vi "read creates channels.vi"(8 "error in":errorcluster, 11 "module configuration in":refnum<class "Scan Engine configuration.lvclass">) -> (0 "error out":errorcluster, 2 "creates channels?":bool, 3 "module configuration out":refnum<class "Scan Engine configuration.lvclass">)   [LabVIEW 2013, in "Scan Engine configuration.lvclass"]
doc: "Provides an interface for determining if a runtime module associated with this configuration is capable of dynamically discovering channels through <b>component runtime interface.lvclass:discover channels.vi</b>. <b>creates channels?</b> defines whether or not a component instance of <b>discover channels.vi</b> will perform any action.NI Tag Bus Module Framework 1.0.2.29\nNI Systems Engineering"
uses:
  Scan Engine configuration.lvclass
  Scan Engine configuration.lvclass/Scan Engine configuration.ctl
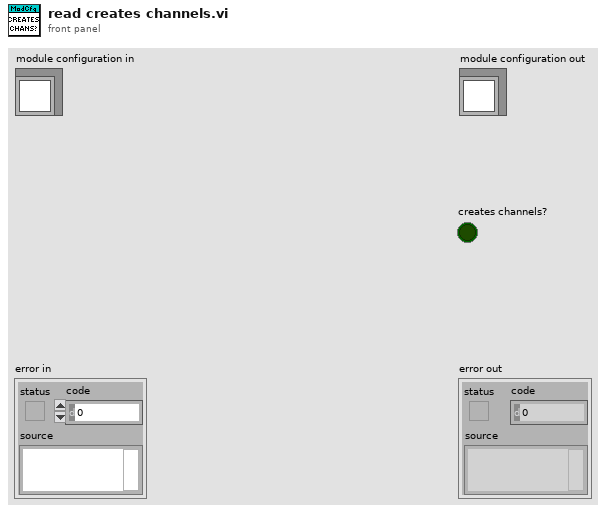
[diagram p1: front panel]
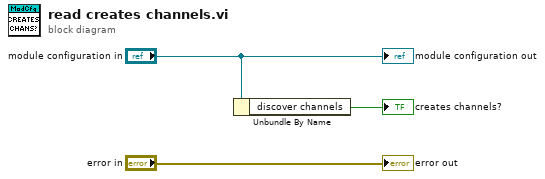
[diagram p0: block diagram]
diagram:
  n1 = Unbundle By Name("module configuration in") -> ("discover channels"=→"creates channels?":bool)
  "error out" <- "error in"
  "module configuration out" <- "module configuration in"
